vi "niScope EX Fetch Forever.vi"() -> ()   [LabVIEW 2024]
uses:
  <instrlib>/niScope/Controls/niScope trigger source.ctl
  <instrlib>/niScope/Configure/Trigger/niScope Configure Trigger Edge.vi
  <instrlib>/niScope/Acquire/Fetch/niScope Fetch Binary 8.vi
panel:
  in  "Simulate?":bool
  out "Waveform from Scope":dbl[](graph)
  in  "Max. Points per Fetch":i32=1000
  in  "Plot Data?":bool=TRUE
  out "Last Points Fetched":i32
  out "Total Points Fetched":i32
  in  "Stop Button":bool
  in  "Channel Name":string="0" caption="Channel(s)"
  in  "Resource Name":refnum<k15>="Dev1" caption="Resource Name(s)"
  in  "Min. Sample Rate":dbl=10000000.0 format="%#_6p"
  in  "Vertical Range (V)":dbl=2.0 format="%_3g"
  # "Overview: Demonstrates using continuous acquisition to fetch an infinite record of data (or until you press stop). \nRequirements: NI-SCOPE\nInstructions: \n1.  Select the appropriate device in the Resource Name(s) control.\n2.  Enter the channels you would like to acquire from in the Channel(s) control.\n3.  Ensure the values entered in the Min Sample Rate, Vertical Range, and Max Points Per Fetch are appropriate.\n4.  Run the VI."
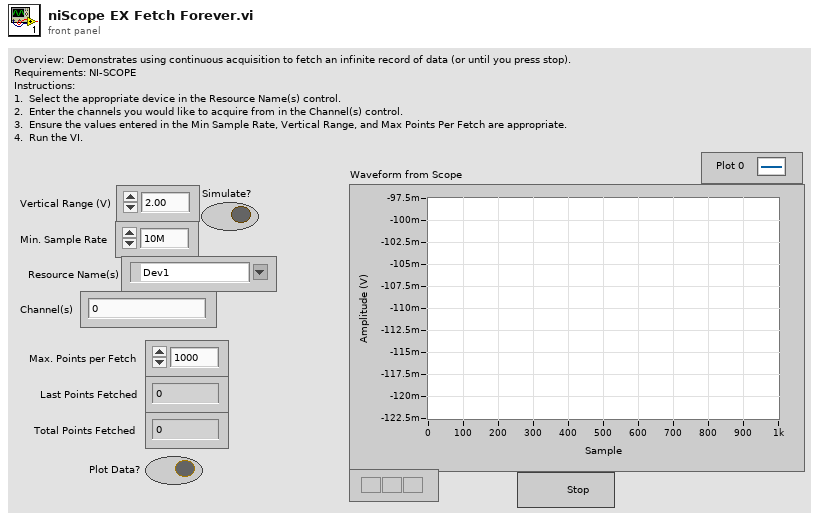
[diagram p1: front panel]
types:
  T1 = typedef "niScope trigger source.ctl" = string
  T2 = cluster{"actualSamples":i32, "absoluteInitialX":dbl, "relativeInitialX":dbl, "xIncrement":dbl, "offset":dbl, "gain":dbl, "reserved1":dbl, "reserved2":dbl}
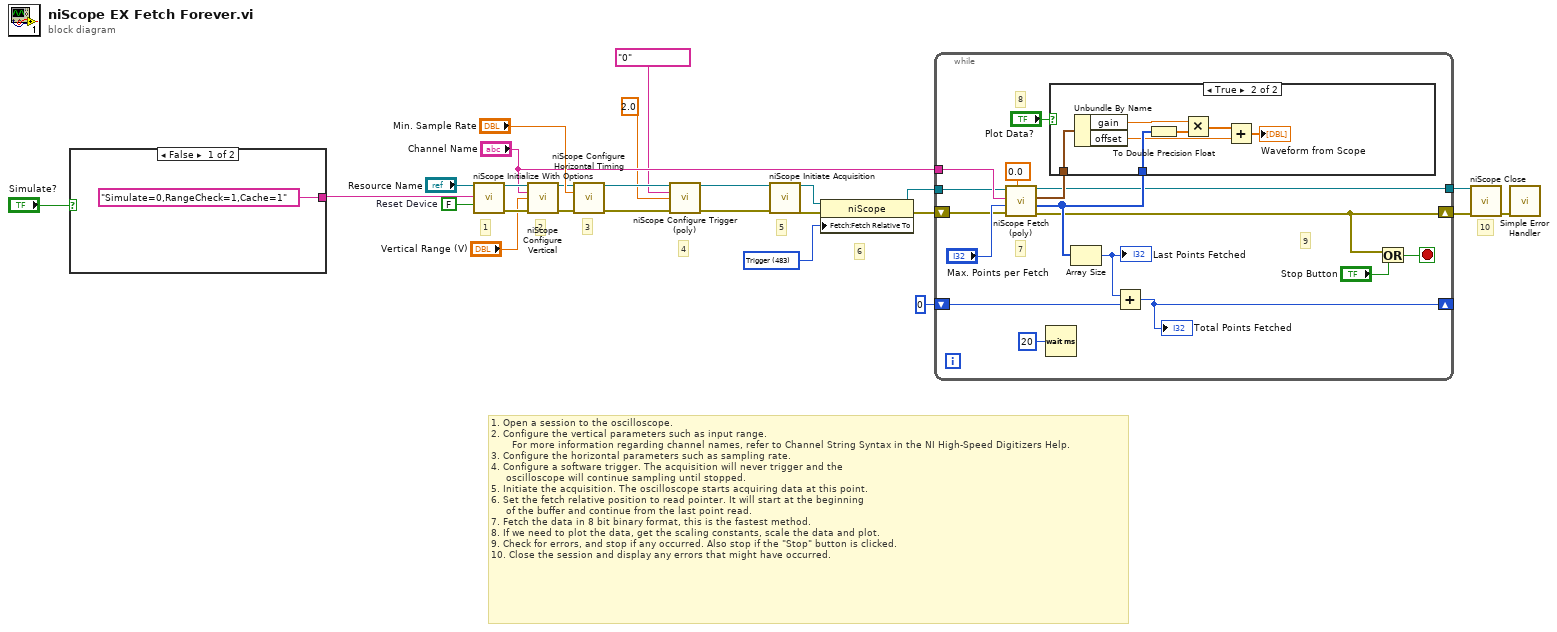
[diagram p0: block diagram]
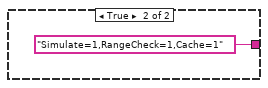
[diagram p2: hidden frame]
diagram:
  w5 = 483 items=["Start"=482, "Trigger"=483, "Pretrigger"=477, "Now"=481, "Read Pointer"=388] ("Fetch:Fetch Relative To")
  w24 = FALSE  # Reset Device
  # "1. Open a session to the oscilloscope.\n2. Configure the vertical parameters such as input range.\n       For more information regarding channel names, refer to Channel String Syntax in the NI High-Speed Digitizers Help.\n3. Configure the horizontal parameters such as sampling rate.\n4. Configure a software trigger. The acquisition will never trigger and the\n     oscilloscope will continue sampling until stopped.\n5. Initiate the acquisition. The oscilloscope starts acquiring data at this point.\n6. Set the fetch relative position to read pointer. It will start at the beginning\n     of the buffer and continue from the last point read.\n7. Fetch the data in 8 bit binary format, this is the fastest method.\n8. If we need to plot the data, get the scaling constants, scale the data and plot.\n9. Check for errors, and stop if any occurred. Also stop if the \"Stop\" button is clicked.\n10. Close the session and display any errors that might have occurred."
  # "10"
  # "6"
  # "5"
  # "4"
  # "3"
  # "2"
  # "1"
  n1 = case shown="False" "Simulate?" {
    tunnel: ["Simulate=0,RangeCheck=1,Cache=1" ("option string") "Simulate=1,RangeCheck=1,Cache=1" ("option string")] -> w3
    frame False {
    }
    frame True {
    }
  }
  n2 = call <instrlib>:"niScope Initialize With Options.vi"("resource name"="Resource Name", "option string"=w3, "reset device"=w24) -> ("instrument handle"=w26:refnum<k15>, "error out"=w25:errorcluster)  [unwired: 11 in]
  n3 = call <instrlib>:"niScope Configure Vertical.vi"("instrument handle"=w26, "channels"="Channel Name", "vertical range"="Vertical Range (V)", "error in"=w25) -> ("instrument handle out"=w16:refnum<k15>, "error out"=w15:errorcluster)  [unwired: 10 in]
  n4 = call <instrlib>:"niScope Configure Horizontal Timing.vi"("instrument handle"=w16, "min sample rate"="Min. Sample Rate", "error in"=w15) -> ("instrument handle out"=w22:refnum<k15>, "error out"=w23:errorcluster)  [unwired: 11 in]
  n5 = call-poly <instrlib>:"niScope Configure Trigger (poly).vi"("instrument handle"=w22, "trigger source"=T1 "0", "trigger level"=2.0, "error in"=w23) -> ("instrument handle out"=w18:refnum<k15>, "error out"=w17:errorcluster)  [unwired: 10 in]
  n6 = call <instrlib>:"niScope Initiate Acquisition.vi"("instrument handle"=w18, "error in"=w17) -> ("instrument handle out"=w10:refnum<k15>, "error out"=w13:errorcluster)  [unwired: 12 in]
  n7 = property class="niScope"(reference=w10, error in=w13, "Fetch:Fetch Relative To"=w5) -> (reference out=w9:refnum<k15>, error out=w8:errorcluster)
  n8 = while {
    shift-left: 0 -> [w44]
    shift-right: [w41] -> _
    tunnel: "Channel Name" -> [w42]
    tunnel: w9 -> [w33]
    tunnel: [w31] -> w6
    shift-right: [w29] -> w7
    shift-left: w8 -> [w32]
    stop <- w43 stop-if-true
    # "9"
    # "8"
    # "7"
    n9 = call-poly <instrlib>:"niScope Fetch (poly).vi"("timeout"=0.0, "error in"=w32, "numSamples"="Max. Points per Fetch", "channels"=w42, "instrument handle"=w33) -> ("error out"=w29:errorcluster, "wfm"=w38:i8[], "wfm info"=w36:T2, "instrument handle out"=w31:refnum<k15>)  [unwired: 3 in]
    n10 = Wait (ms)(milliseconds to wait=u32 20) -> ()  [unwired: 1 out]
    n11 = case shown="True" "Plot Data?" {
      tunnel: w38 -> [_ w50]
      tunnel: w36 -> [_ w51]
      frame False {
      }
      frame True {
        n12 = Unbundle By Name(w51) -> ("gain"=w49:dbl, "offset"=w47:dbl)
        n13 = To Double Precision Float(number=w50) -> (double precision float=w45:dbl[])
        n14 = Multiply(x=w49, y=w45) -> (x*y=w48:dbl[])
        n15 = Add(x=w48, y=w47) -> (x+y=→"Waveform from Scope":dbl[])
      }
    }
    n16 = Array Size(array=w38) -> (size(s)=w37:i32)
    "Last Points Fetched" <- w37
    n17 = Add(x=w37, y=w44) -> (x+y=w41:i32)
    "Total Points Fetched" <- w41
    n18 = Or(x=w29, y="Stop Button") -> (x .or. y?=w43:bool)
  }
  n19 = call <instrlib>:"niScope Close.vi"("instrument handle"=w6, "error in"=w7) -> ("error out"=w12:errorcluster)  [unwired: 13 in]
  n20 = call <vilib>:"Simple Error Handler.vi"("error in (no error)"=w12) -> ()  [unwired: 4 in, 5 out]
